vi "IsLoggedIn.vi"(8 "error in (no error)":errorcluster, 11 "reference in":refnum<class "MES_Local.lvclass">) -> (0 "error out":errorcluster, 1 "OK":bool, 3 "reference in":refnum<class "MES_Local.lvclass">)   [LabVIEW 2022 SP3, in "MES_Local.lvlib" / "MES_Local.lvclass"]
uses:
  MES_Local.lvclass
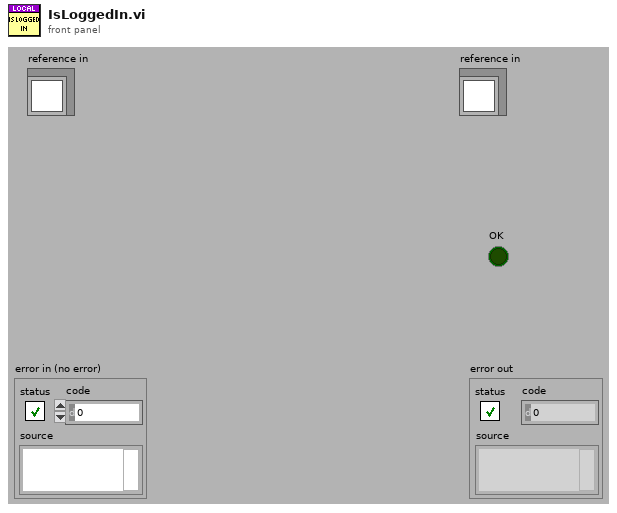
[diagram p1: front panel]
types:
  T1 = typedef "MES_Local.lvlib/MES_Local.lvclass/ObjectAttributes.ctl" = cluster{"Config":T2, "Logged_In?":bool, "AttributeNames":string[], "AttributeWritten":bool[], "ComponentNames":string[], "TestIndex":i32, "TestTag":string[], "Time Stamp":timestamp, "Employee":string, "Resource_Key":string, "Local Spec":path, "Login":refnum<class "Login_Base.lvclass">, "ReportPath":path, "Spec":T3, "StartTime":timestamp, "Role":string}
  T2 = typedef "MES_Local.lvlib/MES_Local.lvclass/Config.ctl" = cluster{"Results_Path":path}
  T3 = typedef "MES_Base.lvlibp/MES_Base.lvclass/Spec.ctl" = cluster{"Header":cluster{"Doctype":string, "Checksum":string, "DriverKey":string, "SpecId":string, "TransactionId":string, "AccountId":string, "SpecName":string, "WorkflowStep":string, "SerialNumber":string, "BatchNumber":string, "Status":enum16{"Pending", "Pass", "Fail"}, "Comment":string, "FirstFail":string, "Employee":string, "LocalMachine":string, "ResourceKey":string, "Date":string, "Time":string, "Duration":string, "DUT Position":i32}, "Components":cluster{"SerialNumber":string, "PartNumber":string, "Revision":string, "BatchNumber":string, "Name":string, "Description":string, "Attached":bool}[], "Attributes":cluster{"Name":string, "Description":string, "DataType":enum16{"NA", "String", "Boolean", "Int", "Dbl"}, "Value":variant, "DisplayFormat":string, "ReadOnly":bool, "Required":bool}[], "Tests":cluster{"Code":string, "Name":string, "Description":string, "Group":string, "IsGroup":bool, "Tag":string, "Method":string, "Parrameter":string, "DataType":enum16{"NA", "String", "Boolean", "Int", "Dbl"}, "Value":variant, "Status":enum16{"Pending", "Pass", "Fail"}, "LimitLo":variant, "LimitHi":variant, "StringMatch":string, "BooleanMatch":bool, "DisplayFormat":string, "Units":string, "TestTime":dbl}[]}
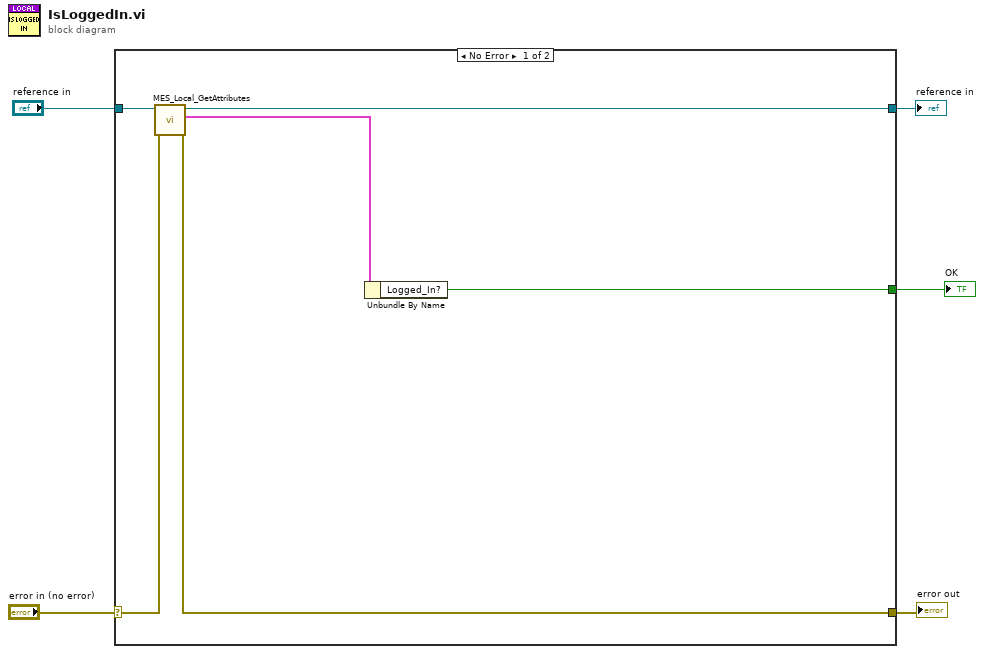
[diagram p0: block diagram]
diagram:
  n1 = case shown="No Error" "error in (no error)" {
    selector: "error in (no error)" -> [w11 w13]
    tunnel: [w9 w13] -> w4
    tunnel: [w7 w12] -> w2
    tunnel: "reference in" -> [w8 w12]
    tunnel: [w6 _] -> w1
    frame No Error {
      n2 = call "MES_Local_GetAttributes.vi"("error in (no error)"=w11, "reference in"=w8) -> ("error out"=w9:errorcluster, "Data"=w10:T1, "reference out"=w7:refnum<class "MES_Local.lvclass">)  [unwired: 6 in, 1 out]
      n3 = Unbundle By Name(w10) -> ("Logged_In?"=w6:bool)
    }
    frame Error {
    }
  }
  "error out" <- w4
  "reference in" <- w2
  "OK" <- w1
